vi "SensorTest.vi"() -> ()   [LabVIEW 2020]
panel:
  out "Waveform Chart 5":dbl(graph)
  out "Waveform Chart 4":dbl(graph)
  out "AI2 2":dbl
  out "AI1 2":dbl
  out "AI0 2":dbl
  out "AI2":dbl
  out "AI1":dbl
  out "AI0":dbl
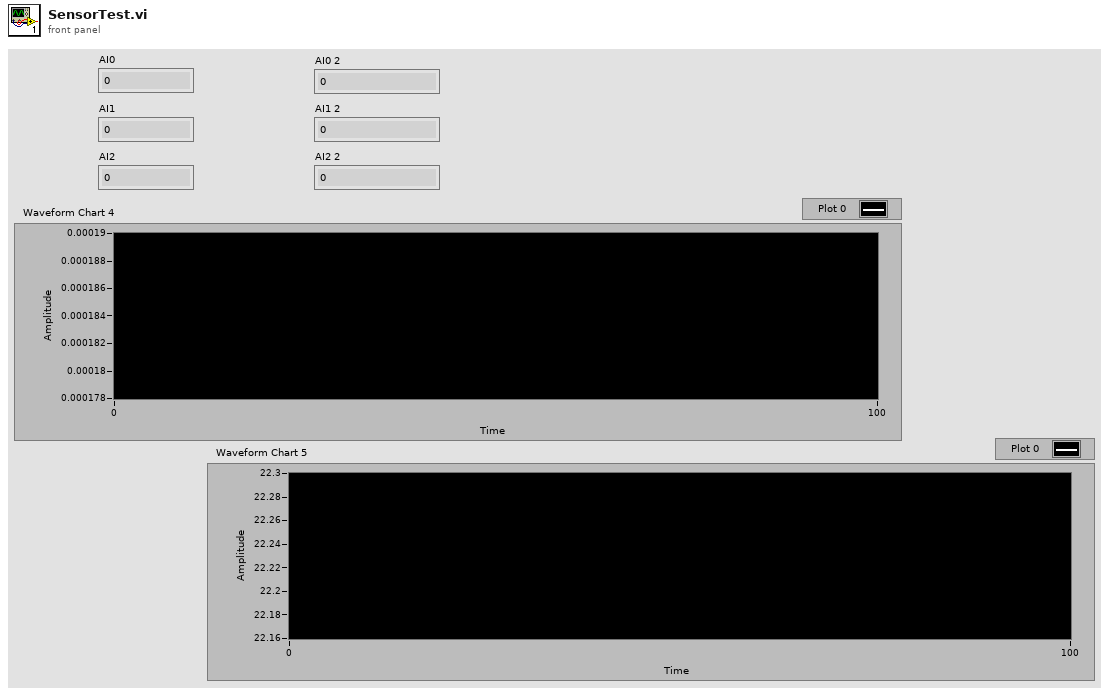
[diagram p1: front panel]
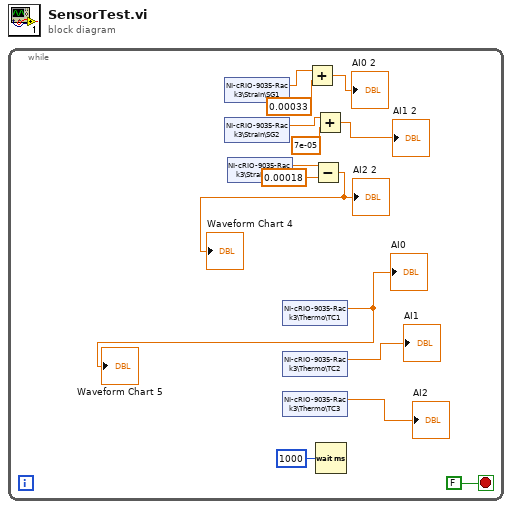
[diagram p0: block diagram]
diagram:
  n1 = while {
    stop <- FALSE stop-if-true
    n2 = shared-variable "NI-cRIO-9035-Rack3\\Strain\\SG1"() -> (w9:dbl)  [unwired: 1 in, 1 out]
    n3 = shared-variable "NI-cRIO-9035-Rack3\\Strain\\SG2"() -> (w5:dbl)  [unwired: 1 in, 1 out]
    n4 = shared-variable "NI-cRIO-9035-Rack3\\Strain\\SG3"() -> (w3:dbl)  [unwired: 1 in, 1 out]
    n5 = shared-variable "NI-cRIO-9035-Rack3\\Thermo\\TC1"() -> (→"AI0" →"Waveform Chart 5":dbl)  [unwired: 1 in, 1 out]
    n6 = shared-variable "NI-cRIO-9035-Rack3\\Thermo\\TC2"() -> (→"AI1":dbl)  [unwired: 1 in, 1 out]
    n7 = shared-variable "NI-cRIO-9035-Rack3\\Thermo\\TC3"() -> (→"AI2":dbl)  [unwired: 1 in, 1 out]
    n8 = Add(x=w9, y=0.00033) -> (x+y=→"AI0 2":dbl)
    n9 = Subtract(x=w3, y=0.00018) -> (x-y=→"AI2 2" →"Waveform Chart 4":dbl)
    n10 = Add(x=w5, y=7e-05) -> (x+y=→"AI1 2":dbl)
    n11 = Wait (ms)(milliseconds to wait=u32 1000) -> ()  [unwired: 1 out]
  }
